vi "CSM - Wait and Post Message.vi"(0 "State":string="API State", 1 "Current Module (\"\" to Generate an ID)":string, 5 "Arguments (\"\")":string, 7 "Target Module":string="Target", 9 "Wait (5000ms)":i32=5000, 11 "Error In (No Error)":errorcluster) -> (10 "Waited (ms)":u32, 15 "error out":errorcluster)   [LabVIEW 2017, in "Communicable State Machine.lvlib"]
doc: "Sends an asynchronous message to the specified CSM module. Since the transmission is asynchronous, this VI does not wait for a reply, and code execution continues immediately after the message is sent. If the CSM module does not exist, this VI waits for the specified timeout duration. If the timeout is exceeded, a timeout error is returned.\n\n\n> [!NOTE] <b>Asynchronous Message</b>\n>\n> An asynchronous message is a type of message. After a CSM sends an asynchronous message, it immediately continues to execute subsequent code without waiting for the callee to complete message processing. Asynchronous messages are divided into Asynchronous Call (`->`) and Asynchronous Call without Reply (`->|`). The only difference is that with an Asynchronous Call without Reply (`->|`), the callee will not return the result to the caller after completing the operation.\n>\n> <b>Errors occurring at the Caller</b>:\n> - If the input target module is `\"\"`, a `NO Target Error` is generated.\n> - If the input module does not exist, a `Target Error` is generated.\n>\n> <b>Caller does not wait for return</b>:\n> - If the caller is a CSM module, it enters the `Async Message Posted` state after sending the message in the Parse State Queue++ VI.\n> - If it is an API call, it continues to execute subsequent code. The API can only send Asynchronous without Reply messages.\n>\n> <b>Return</b>:\n> - <b>If the caller is a CSM module</b>:\n> - Normally, it enters the `Async Response` state to handle the return. If an error occurs at the callee, this information is still the result of the message. It is handled in the `Async Response` state, and this error information can be obtained from Additional Information.\n> - If an error occurs at the caller, it causes the CSM state machine to enter the `Error Handler` module to handle the error.\n> - There is no return if the API can only send Asynchronous without Reply messages.\n\n\n> [!NOTE] <b>CSM Message Target Module Description</b>\n>\n> In Normal Mode, the target module for a CSM message is the specified module name. \n> System-level modules start with a `.` in their name. The target module for a CSM message includes the `.` in the name. For example, if the requested module name is `.System`, the target module for the CSM message is `.System`.\n> In Worker Mode, the target module for a CSM message can only be the overall module name, not the node name. For example, if the requested module name is `Worker#`, the target module for the CSM message is `Worker`. \n> In Chain of Responsibility Mode, the target module for a CSM message can only be the overall module name, not the node name. For example, if the requested module name is `Chain$1`, the target module for the CSM message is `Chain`.\n\n\n-- <b>Controls</b> --\n- <b>Current Module (\"\" to Generate an ID)</b>: Name of the current module. If empty, a temporary ID is generated for debugging purposes to identify the location.\n- <b>State</b>: Message string.\n- <b>Arguments (\"\")</b>: Message arguments.\n- <b>Target Module</b>: Name of the target module.\n- <b>Wait (5000ms)</b>: Timeout duration for waiting. The default is 5000 ms.\n\n-- <b>Indicators</b> --\n- <b>Waited (ms)</b>: Time elapsed while waiting."
uses:
  Communicable State Machine.lvlib
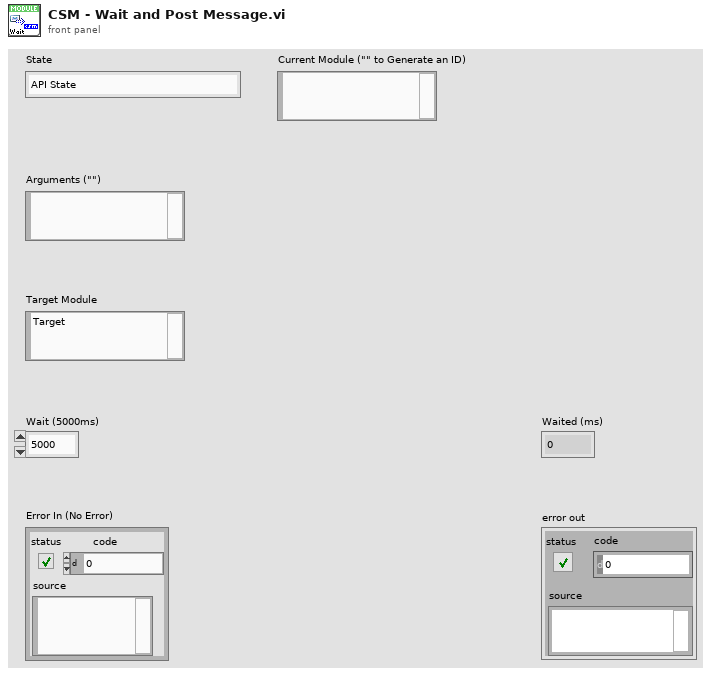
[diagram p1: front panel]
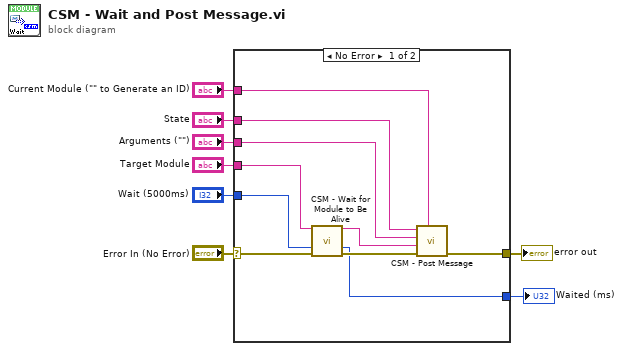
[diagram p0: block diagram]
diagram:
  n1 = case shown="No Error" "Error In (No Error)" {
    selector: "Error In (No Error)" -> [w12 w19]
    tunnel: "State" -> [w17 _]
    tunnel: [w15 w19] -> w6
    tunnel: "Arguments (\"\")" -> [w16 _]
    tunnel: "Target Module" -> [w13 _]
    tunnel: "Current Module (\"\" to Generate an ID)" -> [w18 _]
    tunnel: "Wait (5000ms)" -> [w14 _]
    tunnel: [w9 _] -> w1
    frame No Error {
      n2 = call "CSM - Wait for Module to Be Alive.vi"("CSM Name"=w13, "Wait (5000 ms)"=w14, "error in (no error)"=w12) -> ("CSM Name (Dup)"=w10:string, "Waited (ms)"=w9:u32, "error out"=w11:errorcluster)  [unwired: 10 in]
      n3 = call "CSM - Post Message.vi"("Current Module (\"\" to Generate an ID)"=w18, "Error In (No Error)"=w11, "Target Module"=w10, "Arguments (\"\")"=w16, "State"=w17) -> ("error out"=w15:errorcluster)  [unwired: 6 in]
    }
    frame Error {
    }
  }
  "error out" <- w6
  "Waited (ms)" <- w1
